vi "XMarkersToWL.vi"(1 "1:1024":i32[](array[numeric]), 2 "CenterWL":ext) -> (0 "px2nm(CenterWL, 1:1024)":dbl[](array[numeric]))   [LabVIEW 2019]
panel:
  out "A":dbl
  out "B":dbl
  out "C":ext
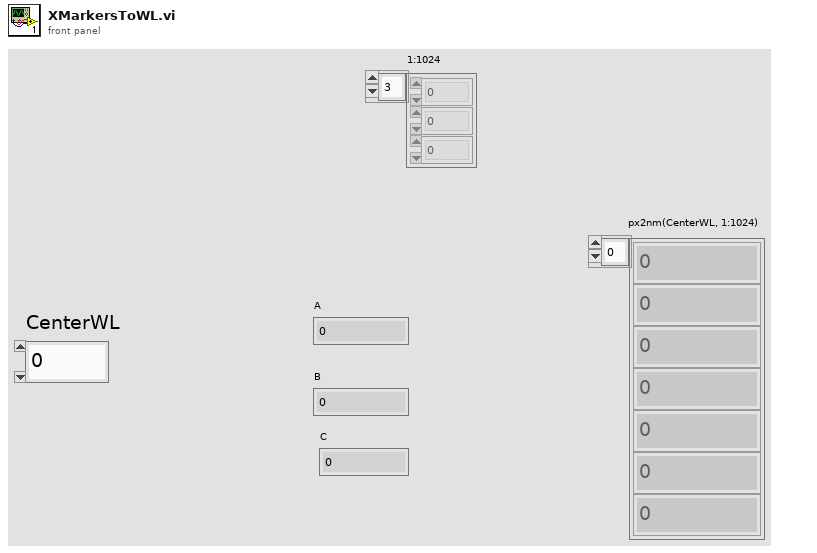
[diagram p1: front panel]
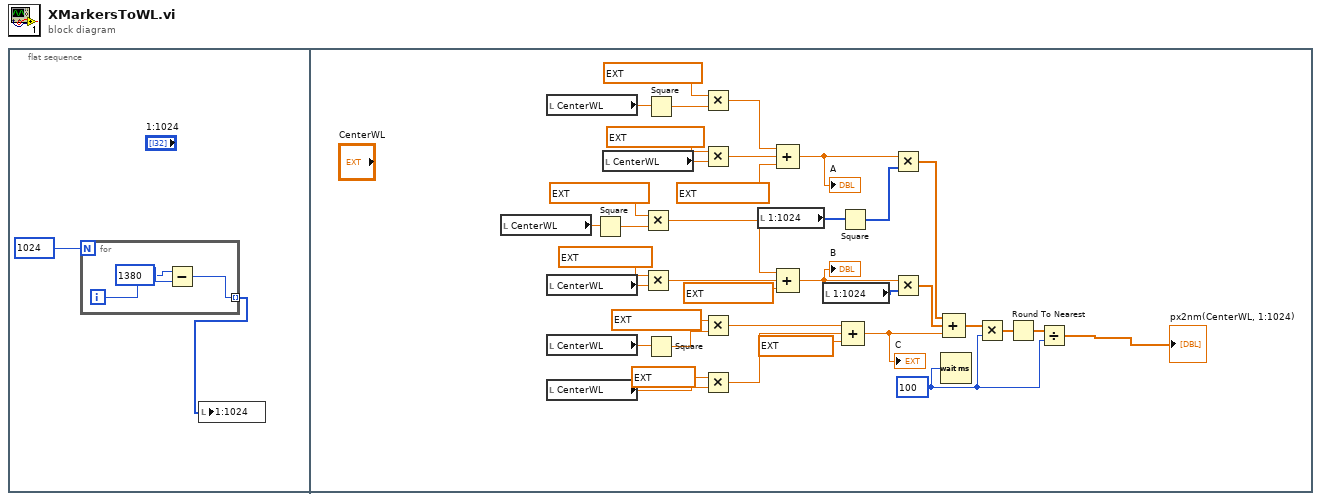
[diagram p0: block diagram]
diagram:
  n1 = flat-sequence {
    frame #0 {
      n2 = for {
        N: 1024 -> [_]
        tunnel: [w3] -> w1 mode=indexing
        i -> [w5]
        n3 = Subtract(x=1380, y=w5) -> (x-y=w3:i32)
      }
      n4 = local write "1:1024"(w1) -> ()
    }
    frame #1 {
      w41 = 100
      n5 = local read "CenterWL"() -> (w25:ext)
      n6 = local read "CenterWL"() -> (w40:ext)
      n7 = local read "CenterWL"() -> (w28:ext)
      n8 = local read "CenterWL"() -> (w24:ext)
      n9 = local read "CenterWL"() -> (w21:ext)
      n10 = Square(x=w25) -> (x^2=w26:ext)
      n11 = local read "CenterWL"() -> (w37:ext)
      n12 = Multiply(x=ext -2.725807e-8, y=w26) -> (x*y=w30:ext)
      n13 = Multiply(x=ext -6.1133820000000000002e-8, y=w28) -> (x*y=w31:ext)
      n14 = Square(x=w40) -> (x^2=w39:ext)
      n15 = Square(x=w24) -> (x^2=w23:ext)
      n16 = Multiply(x=ext 4.049914e-13, y=w39) -> (x*y=w35:ext)
      n17 = Multiply(x=ext -1.668507e-9, y=w37) -> (x*y=w34:ext)
      n18 = Multiply(x=ext 0.00001387984, y=w23) -> (x*y=w19:ext)
      n19 = Multiply(x=ext 1.00043999999999999996, y=w21) -> (x*y=w18:ext)
      n20 = local read "1:1024"() -> (w8:i32[])
      n21 = Compound Arithmetic op=ADD(w35, w34, ext -6.6831310000000000002e-7) -> (w42:ext)
      "A" <- w42
      n22 = Compound Arithmetic op=ADD(w30, w31, ext 0.04387259) -> (w13:ext)
      "B" <- w13
      n23 = local read "1:1024"() -> (w7:i32[])
      n24 = Square(x=w8) -> (x^2=w14:i32[])
      n25 = Compound Arithmetic op=ADD(w19, w18, ext -22.28139) -> (w12:ext)
      "C" <- w12
      n26 = Multiply(x=w42, y=w14) -> (x*y=w15:ext[])
      n27 = Multiply(x=w13, y=w7) -> (x*y=w16:ext[])
      n28 = Wait (ms)(milliseconds to wait=w41) -> ()  [unwired: 1 out]
      n29 = Compound Arithmetic op=ADD(w15, w16, w12) -> (w11:ext[])
      n30 = Multiply(x=w11, y=w41) -> (x*y=w10:ext[])
      n31 = Round To Nearest(number=w10) -> (nearest integer value=w9:ext[])
      n32 = Divide(x=w9, y=w41) -> (x/y=→"px2nm(CenterWL, 1:1024)":ext[])
    }
  }
